vi "main v2.vi"() -> ()   [LabVIEW 2018]
uses:
  project/type defs/test keypad luster.ctl
  <vilib>/Instr/_visa.llb/VISA Configure Serial Port (Instr).vi
  type defs/Pelco_D_cmd.vi
  <vilib>/NI/Modbus Library/API/Wrapper/Create Serial Master.vi
  <vilib>/NI/Modbus Library/API/Master/Modbus Master.lvclass
  <vilib>/NI/Modbus Library/API/Wrapper/API Main.lvlib
panel:
  in  "autoFocus":bool
  out "Remote TILT":dbl format="%#_6f"
  out "Remote PAN":dbl format="%#_6f"
  in  "Client Closed":string="The client VI closed the connection."
  out "Reset status":bool
  in  "enable":bool=TRUE
  out "tilt":dbl
  out "pan":dbl
  in  "pan_right_limit(-10) 2":dbl=-20.0
  in  "pan left_limit(20) 2":dbl=20.0
  in  "tilt_down_limit(-10)":dbl=-10.0
  in  "tilt_up_limit(20)":dbl=20.0
  in  "delta tilt/sec":dbl=0.1 format="%#.13f"
  in  "delta pan/sec":dbl=0.1 format="%#.13f"
  out "launcher.compass":dbl format="%.1f"
  out "launcher.tilt":dbl format="%.1f"
  out "launcher.pan":dbl format="%.1f"
  out "magnification":string
  in  "get magnification":bool
  in  "cam default":bool
  in  "reset":bool
  out "Sync Status":bool
  out "keypad cmd":string
  out "CAM.tilt":dbl format="%#.2g"
  out "CAM.pan":dbl format="%.2f"
  in  "read tilt":bool
  in  "read pan":bool
  in  "close com":bool
  in  "open com":bool
  in  "stop":bool
  # "Launcher"
  # "Camera"
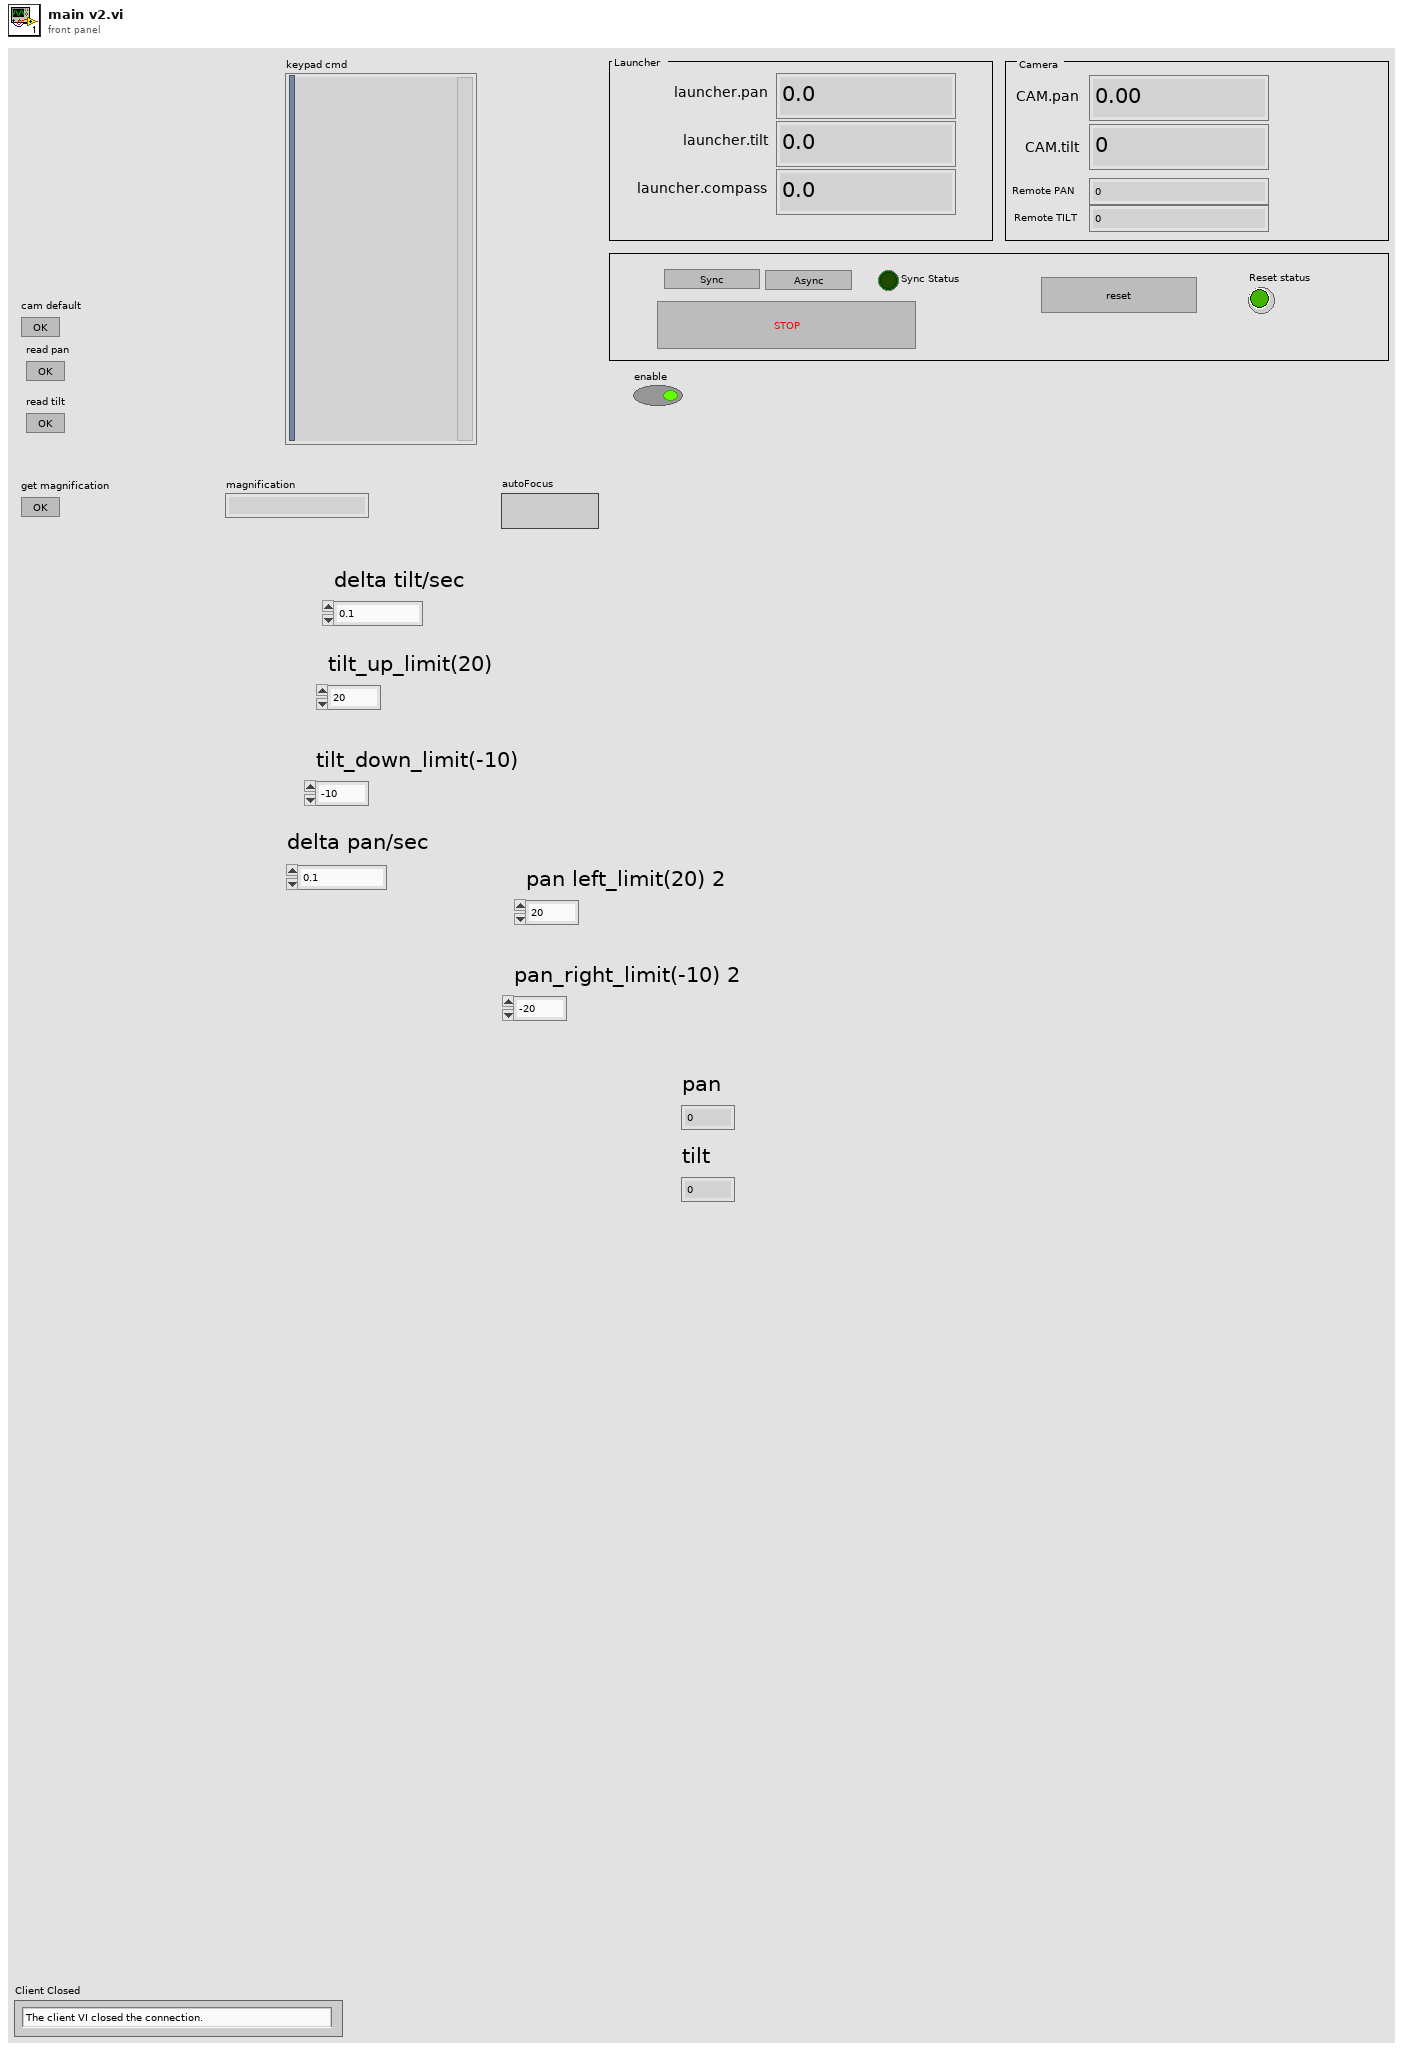
[diagram p1: front panel]
types:
  T1 = cluster{"launcher_pan":i16, "launcher_tilt":i16, "launcher_pan_leftLimit":i16, "launcher_pan_rightLimit":i16, "launcher_tilt_downLimit":i16, "launcher_tilt_upLimit":i16, "launcher_PLClink":i16, "launcher_PLCstatus":i16, "CAM_pan":i16, "CAM_tilt":i16}
  T2 = typedef "test keypad luster.ctl" = cluster{"cmd":string, "keypad cmd":variant}
  T3 = typedef "App Cluster.ctl" = cluster{"Hadware":cluster{"SPIM7.Keypad":refnum<visa-resource-name>, "SPIM7.CAM":refnum<visa-resource-name>, "PLC":refnum<visa-resource-name>, "Tester":refnum<visa-resource-name>, "ND3Comm":refnum<visa-resource-name>}, "Offset":cluster{"Pan":cluster{"a":dbl, "b":dbl}, "Tilt":cluster{"a":dbl, "b":dbl}}}
  T4 = cluster{"quit":refnum<user-event>, "read tilt":refnum<user-event>, "read pan":refnum<user-event>}
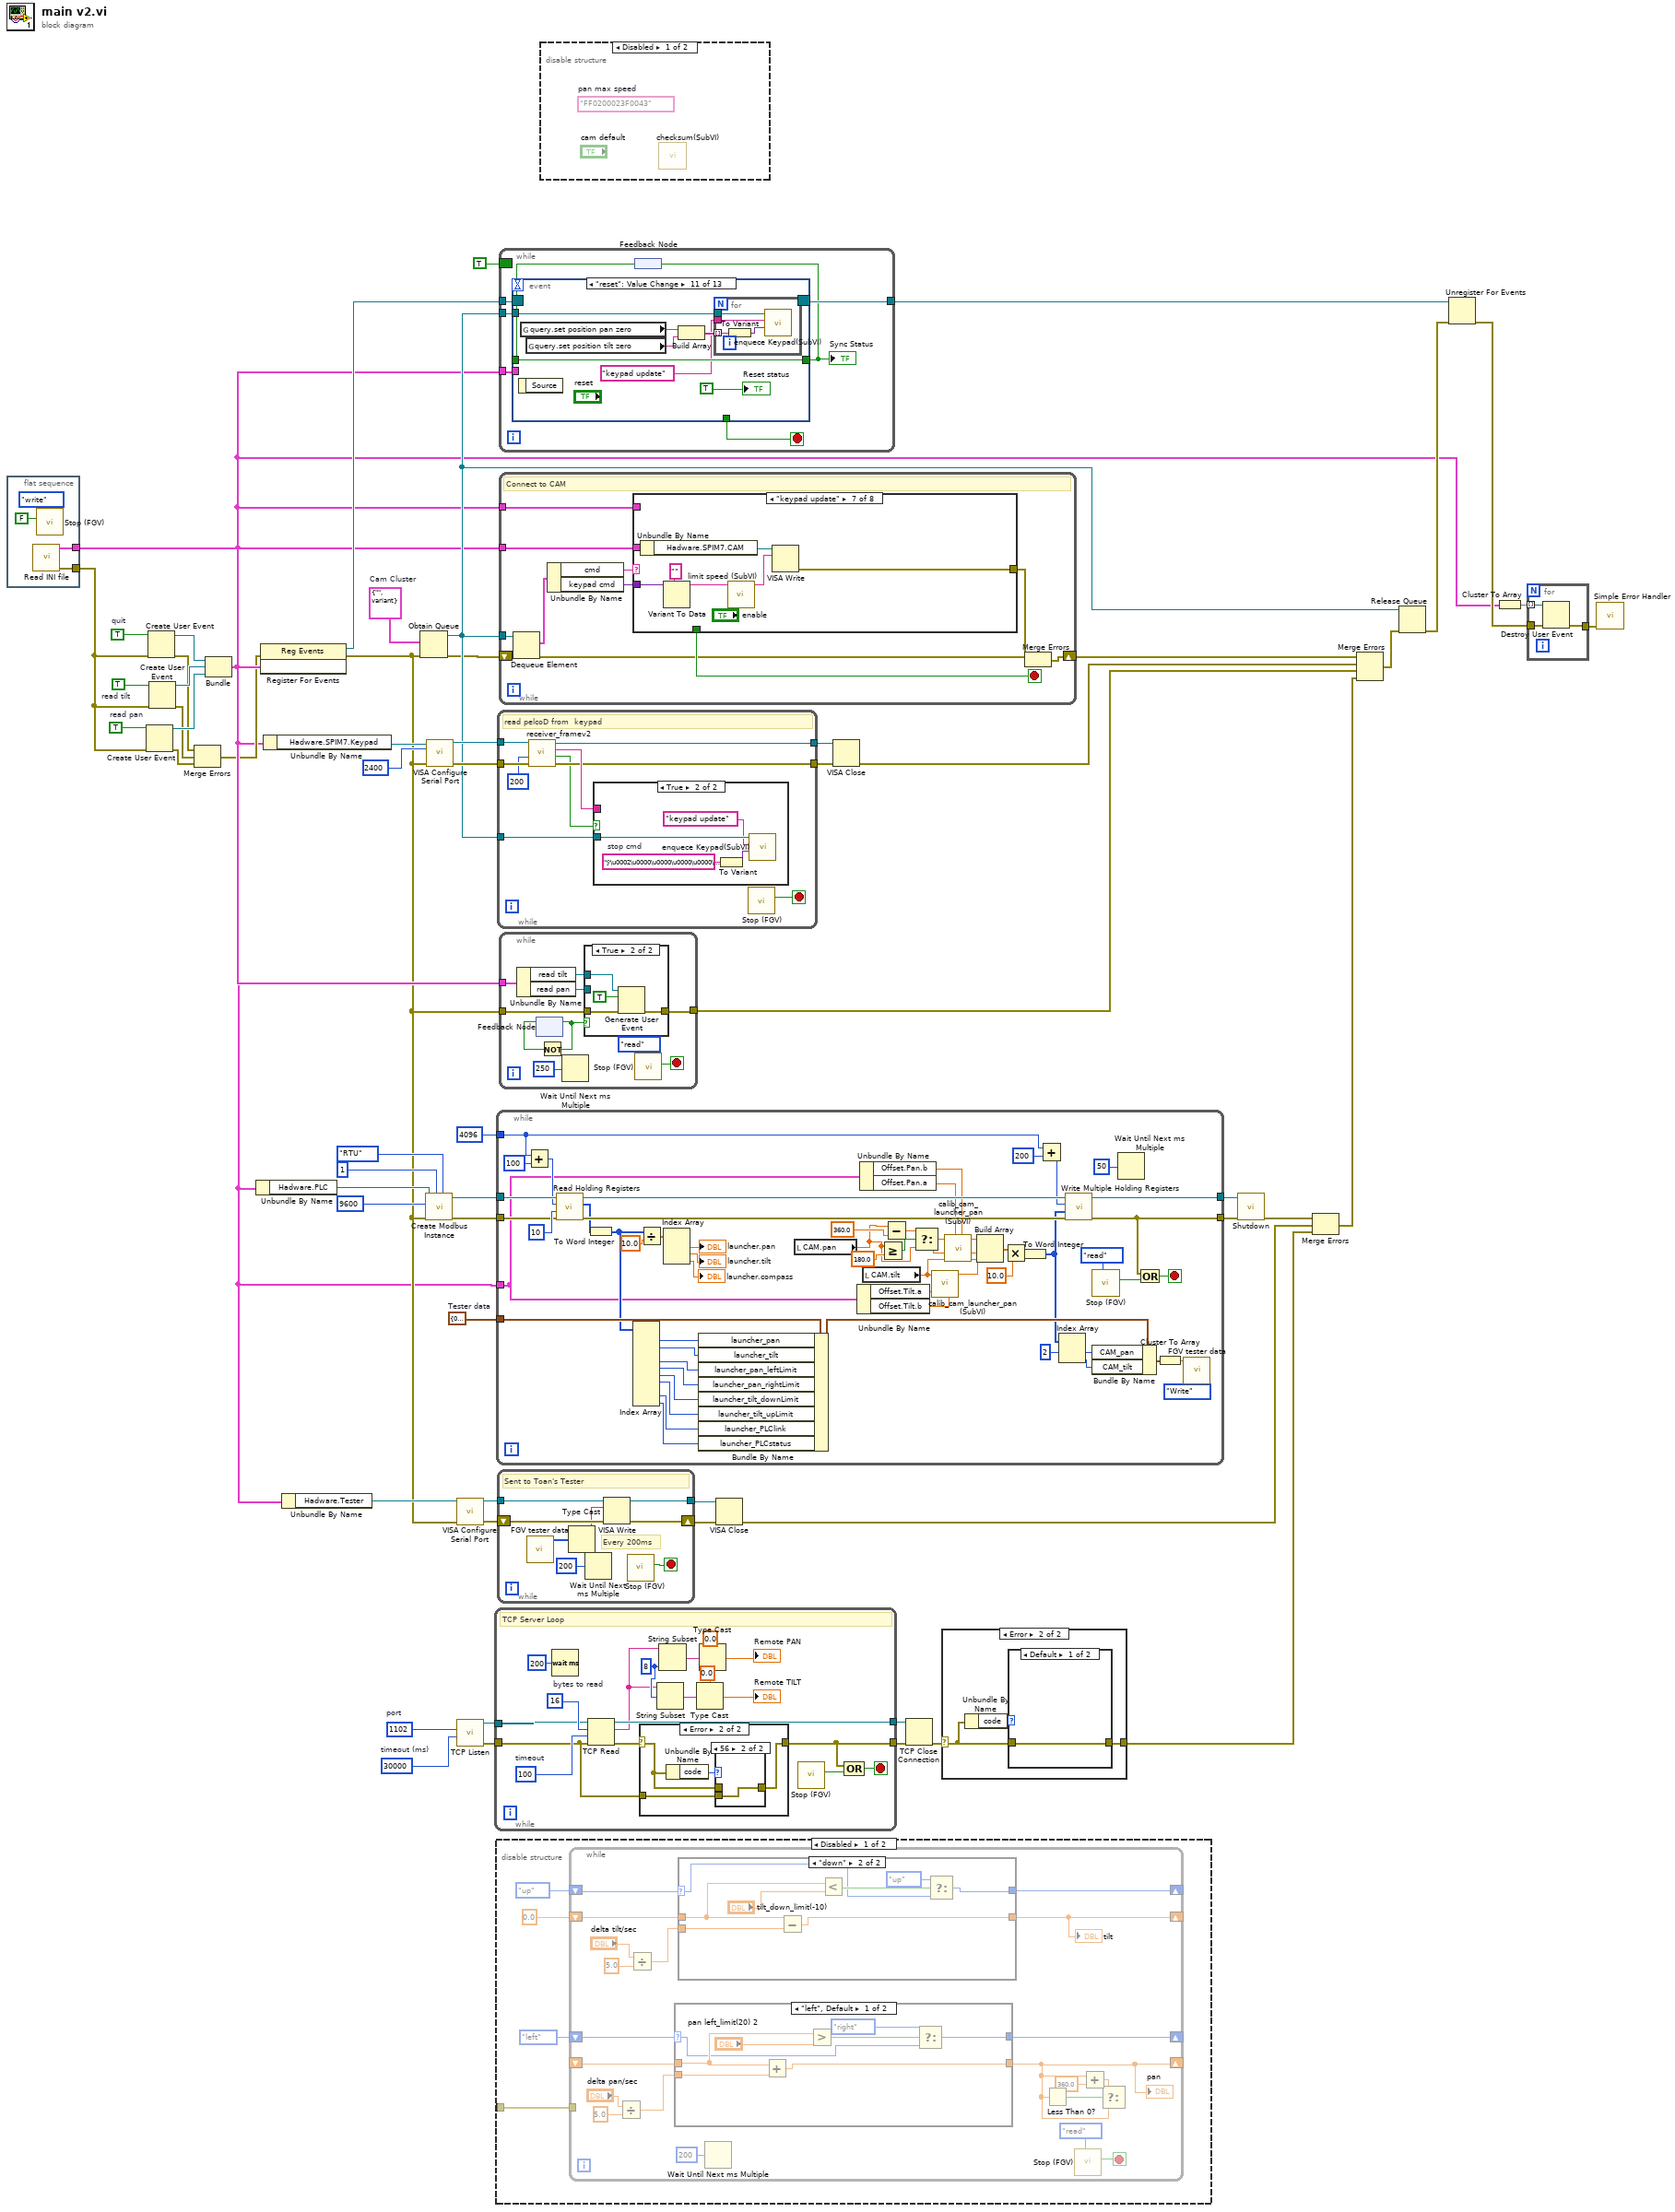
[diagram p0: block diagram]
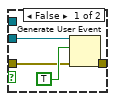
[diagram p2: hidden frame]
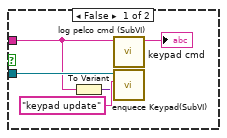
[diagram p3: hidden frame]
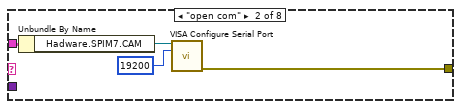
[diagram p5: hidden frame]
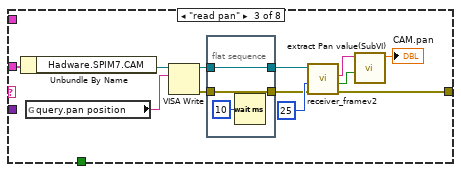
[diagram p6: hidden frame]
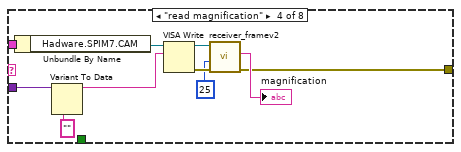
[diagram p7: hidden frame]
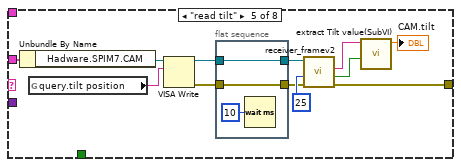
[diagram p8: hidden frame]
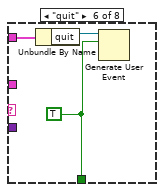
[diagram p9: hidden frame]
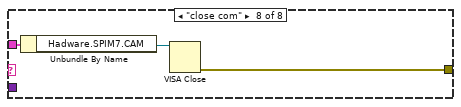
[diagram p10: hidden frame]
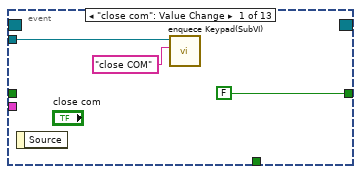
[diagram p11: hidden frame]
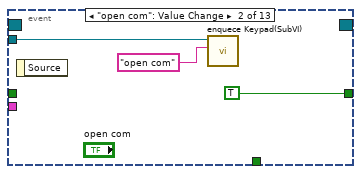
[diagram p12: hidden frame]
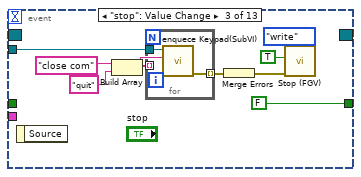
[diagram p13: hidden frame]
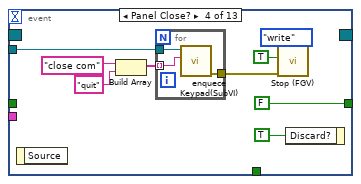
[diagram p14: hidden frame]
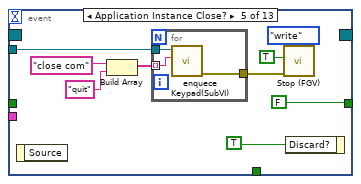
[diagram p15: hidden frame]
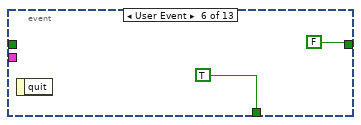
[diagram p16: hidden frame]
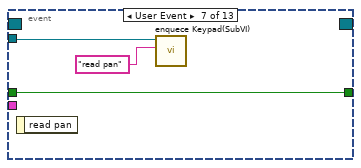
[diagram p17: hidden frame]
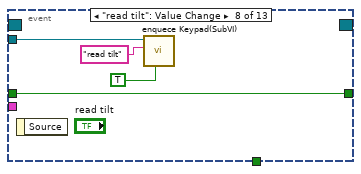
[diagram p18: hidden frame]
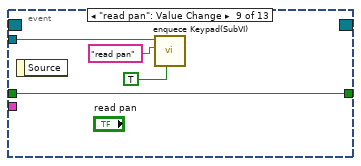
[diagram p19: hidden frame]
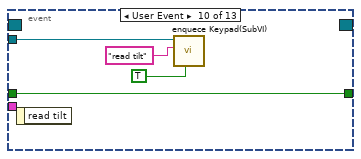
[diagram p20: hidden frame]
diagram:
  w27 = T1 {"launcher_pan"=0, "launcher_tilt"=0, "launcher_pan_leftLimit"=0, "launcher_pan_rightLimit"=0, "launcher_tilt_downLimit"=0, "launcher_tilt_upLimit"=0, "launcher_PLClink"=0, "launcher_PLCstatus"=0, "CAM_pan"=0, "CAM_tilt"=0}  # Tester data
  w13 = u16 1102  # port
  w14 = 30000  # timeout (ms)
  w47 = TRUE  # read pan
  w48 = TRUE  # read tilt
  w60 = TRUE  # quit
  w56 = T2 {"cmd"="", "keypad cmd"=variant(refnum<visa-resource-name> "")}  # Cam Cluster
  n1 = flat-sequence {
    tunnel: [w61] -> w41
    tunnel: [w62] -> w2
    frame #0 {
      n2 = call "Read INI file.vi"() -> ("error out"=w61:errorcluster, "App Cluster out"=w62:T3)  [unwired: 10 in]
      n3 = call "Stop (FGV).vi"("Enum(read)"=enum16{"write", "read"}."write" ("Enum"), "Stop in"=FALSE ("Boolean")) -> ()  [unwired: 8 in, 2 out]
    }
  }
  n4 = Create User Event(user event datatype=w47, error in=w41) -> (user event=w44:refnum<user-event>, error out=w8:errorcluster)
  n5 = Create User Event(user event datatype=w60, error in=w41) -> (user event=w46:refnum<user-event>, error out=w10:errorcluster)
  n6 = Create User Event(user event datatype=w48, error in=w41) -> (user event=w45:refnum<user-event>, error out=w9:errorcluster)
  n7 = Merge Errors(w10, w9, w8) -> (w7:errorcluster)
  n8 = Bundle("quit"=w46, "read tilt"=w45, "read pan"=w44) -> (w36:T4)  [unwired: 1 in]
  n9 = Unbundle By Name(w2) -> ("Hadware.PLC"=w5:refnum<visa-resource-name>)
  n10 = register-events(error in=w7, w36) -> (reference out=w59:refnum<event-registration>, error out=w3:errorcluster)  [unwired: 1 in]
  n11 = Unbundle By Name(w2) -> ("Hadware.SPIM7.Keypad"=w6:refnum<visa-resource-name>)
  n12 = Unbundle By Name(w2) -> ("Hadware.Tester"=w4:refnum<visa-resource-name>)
  n13 = Obtain Queue(element data type=w56, error in (no error)=w3) -> (queue out=w50:refnum<queue>, error out=w37:errorcluster)  [unwired: 3 in, 1 out]
  n14 = call-poly <vilib>:"Create Modbus Instance.vi"("serial type"=enum16{"RTU", "ASCII"}."RTU", "unit ID"=u8 1, "error in"=w3, "baud rate"=u32 9600, "VISA resource name"=w5) -> ("error out"=w30:errorcluster, "serial master instance"=w31:refnum<class "Modbus Master.lvclass">)  [unwired: 5 in]
  n15 = call-poly "VISA Configure Serial Port"("VISA resource name"=w6, "baud rate (9600)"=u32 2400, "error in (no error)"=w3) -> ("VISA resource name out"=w54:refnum<visa-resource-name>, "error out"=w53:errorcluster)  [unwired: 11 in]
  n16 = call-poly "VISA Configure Serial Port"("VISA resource name"=w4, "error in (no error)"=w3) -> ("VISA resource name out"=w26:refnum<visa-resource-name>, "error out"=w25:errorcluster)  [unwired: 12 in]
  n17 = call <vilib>:"TCP Listen.vi"("timeout ms (wait forever: -1)"=w14, "port"=w13) -> ("error out"=w15:errorcluster, "connection ID"=w16:refnum<k5>)  [unwired: 5 in, 3 out]
  n18 = while {
    tunnel: [w76] -> w18
    tunnel: [w79] -> w19
    tunnel: w16 -> [w75]
    tunnel: w15 -> [w74]
    stop <- w81 stop-if-true
    w70 = 8 ("length (rest)")
    w78 = 100  # timeout
    w80 = 16  # bytes to read
    # "TCP Server Loop"
    n19 = Wait (ms)(milliseconds to wait=u32 200) -> ()  [unwired: 1 out]
    n20 = TCP Read(connection ID=w75, bytes to read=w80, error in (no error)=w74, 9:w78) -> (connection ID out=w79:refnum<k5>, data out=w65:string, error out=w77:errorcluster)  [unwired: 1 out]
    n21 = case shown="Error" w77 {
      selector: w77 -> [w83 w86]
      tunnel: [w83 w84] -> w76
      tunnel: w74 -> [_ w85]
      frame No Error {
      }
      frame Error {
        n22 = Unbundle By Name(w86) -> ("code"=w87:i32)
        n23 = case shown="56" w87 {
          tunnel: w86 -> [w88 _]
          tunnel: w85 -> [_ w89]
          tunnel: [w88 w89] -> w84
          frame Default {
          }
          frame 56 {
          }
        }
      }
    }
    n24 = String Subset(string=w65, offset (0)=w70) -> (substring=w68:string)  [unwired: 1 in]
    n25 = String Subset(string=w65, length (rest)=w70) -> (substring=w72:string)  [unwired: 1 in]
    n26 = Type Cast(type=0.0, x=w68) -> (*(type *) &x=→"Remote TILT":dbl)
    n27 = Type Cast(type=0.0, x=w72) -> (*(type *) &x=→"Remote PAN":dbl)
    n28 = call "Stop (FGV).vi"() -> ("Stop out"=w66:bool)  [unwired: 10 in, 1 out]
    n29 = Compound Arithmetic op=OR(w76, w66) -> (w81:bool)
  }
  n30 = while {
    tunnel: u16 4096 -> [w139]
    tunnel: w31 -> [w145]
    tunnel: w30 -> [w141]
    tunnel: [w131] -> w28
    tunnel: [w133] -> w29
    tunnel: w27 -> [w113]
    tunnel: w2 -> [w92]
    stop <- w129 stop-if-true
    n31 = Add(x=w139, y=u16 100) -> (x+y=w143:u16)
    n32 = call-dynamic "Read Holding Registers.vi"("error in"=w141, "number of inputs"=u16 10, "starting address"=w143, "Modbus master in"=w145) -> ("error out"=w134:errorcluster, "register values"=w128:u16[], "Modbus master out"=w136:refnum<class "Modbus Master.lvclass">)  [unwired: 5 in]
    n33 = To Word Integer(number=w128) -> (16bit integer=w111:i16[])
    n34 = Index Array(array=w111) -> (element #1=w110:i16, element #2=w109:i16, element #4=w108:i16, element #5=w107:i16, element #6=w106:i16, element #7=w105:i16, element #9=w104:i16, element #10=w103:i16)  [unwired: 10 in, 2 out]
    n35 = Divide(x=w111, y=10.0) -> (x/y=w124:dbl[])
    n36 = Index Array(array=w124) -> (element #1=→"launcher.pan":dbl, element #2=→"launcher.tilt":dbl, element #3=→"launcher.compass":dbl)  [unwired: 3 in]
    n37 = Bundle By Name(cluster=w113, "launcher_pan"=w110, "launcher_tilt"=w109, "launcher_pan_leftLimit"=w108, "launcher_pan_rightLimit"=w107, "launcher_tilt_downLimit"=w106, "launcher_tilt_upLimit"=w105, "launcher_PLClink"=w104, "launcher_PLCstatus"=w103) -> (w102:T1)
    n38 = local read "CAM.pan"() -> (w118:dbl)
    n39 = Unbundle By Name(w92) -> ("Offset.Tilt.a"=w91:dbl, "Offset.Tilt.b"=w90:dbl)
    n40 = Unbundle By Name(w92) -> ("Offset.Pan.b"=w94:dbl, "Offset.Pan.a"=w93:dbl)
    n41 = local read "CAM.tilt"() -> (w114:dbl)
    n42 = Greater Or Equal?(x=w118, y=180.0) -> (x >= y?=w121:bool)
    n43 = Subtract(x=w118, y=360.0) -> (x-y=w120:dbl)
    n44 = Select(t=w120, s=w121, f=w118) -> (s? t:f=w115:dbl)
    n45 = call "calib_cam_launcher_pan (SubVI).vi"("b"=w90, "a"=w91, "x"=w114) -> ("y"=w116:dbl)  [unwired: 8 in]
    n46 = call "calib_cam_launcher_pan (SubVI).vi"("b"=w94, "a"=w93, "x"=w115) -> ("y"=w117:dbl)  [unwired: 8 in]
    n47 = Build Array(w117, w116, w115, w114) -> (w138:dbl[])
    n48 = Multiply(x=w138, y=10.0) -> (x*y=w112:dbl[])
    n49 = To Word Integer(number=w112) -> (16bit integer=w101:i16[])
    n50 = Add(x=w139, y=u16 200) -> (x+y=w135:u16)
    n51 = Index Array(array=w101, index #1=2 ("index")) -> (element #1=w99:i16, element #2=w98:i16)  [unwired: 1 in]
    n52 = call-dynamic "Write Multiple Holding Registers.vi"("error in"=w134, "registers to write"=w101, "starting address"=w135, "Modbus master in"=w136) -> ("error out"=w131:errorcluster, "Modbus master out"=w133:refnum<class "Modbus Master.lvclass">)  [unwired: 6 in]
    n53 = Bundle By Name(cluster=w102, "CAM_pan"=w99, "CAM_tilt"=w98) -> (w96:T1)
    n54 = call "Stop (FGV).vi"("Enum(read)"=enum16{"write", "read"}."read" ("Enum")) -> ("Stop out"=w130:bool)  [unwired: 9 in, 1 out]
    n55 = Wait Until Next ms Multiple(millisecond multiple=u32 50) -> ()  [unwired: 1 out]
    n56 = Or(x=w131, y=w130) -> (x .or. y?=w129:bool)
    n57 = Cluster To Array(cluster=w96) -> (array=w95:i16[])
    n58 = call "FGV tester data.vi"("Enum(read)"=enum16{"Write", "Read"}."Write" ("Enum"), "data in"=w95) -> ()  [unwired: 9 in, 1 out]
  }
  n59 = disable-structure shown="Disabled" {
    disable-tunnel: _ -> [w147 _]
    frame Disabled {
      n60 = while {
        shift-right: [w162] -> _
        shift-left: 0.0 -> [w166]
        shift-right: [w157] -> _
        shift-left: _ -> [w164]
        shift-right: [w165] -> _
        shift-left: enum16{"up", "down"}."up" -> [w167]
        shift-right: [w161] -> _
        shift-left: enum16{"left", "right"}."left" -> [w163]
        tunnel: w147 -> [_]
        stop <- w168 stop-if-true
        n61 = Divide(x="delta pan/sec", y=5.0) -> (x/y=w154:dbl)
        n62 = Divide(x="delta tilt/sec", y=5.0) -> (x/y=w151:dbl)
        n63 = case shown="\"left\", Default" w163 {
          selector: w163 -> [w173 w181]
          tunnel: w154 -> [w178 w186]
          tunnel: w164 -> [w176 w184]
          tunnel: [w177 w179] -> w157
          tunnel: [w172 w182] -> w161
          frame "left", Default {
            n64 = Add(x=w176, y=w178) -> (x+y=w177:dbl)
            n65 = Greater?(x=w176, y="pan left_limit(20) 2") -> (0:w174:bool)
            n66 = Select(t=enum16{"left", "right"}."right", s=w174, f=w173) -> (s? t:f=w172:enum16{"left", "right"})
          }
          frame "right" {
            n67 = Subtract(x=w184, y=w186) -> (x-y=w179:dbl)
            n68 = Less?(x=w184, y="pan_right_limit(-10) 2") -> (x < y?=w183:bool)
            n69 = Select(t=enum16{"left", "right"}."left", s=w183, f=w181) -> (s? t:f=w182:enum16{"left", "right"})
          }
        }
        "pan" <- w157
        n70 = case shown="\"down\"" w167 {
          selector: w167 -> [w188 w195]
          tunnel: w151 -> [w194 w202]
          tunnel: w166 -> [w192 w199]
          tunnel: [w193 w201] -> w162
          tunnel: [w187 w197] -> w165
          frame "up", Default {
            n71 = Add(x=w192, y=w194) -> (x+y=w193:dbl)
            n72 = Greater?(x=w192, y="tilt_up_limit(20)") -> (0:w190:bool)
            n73 = Select(t=enum16{"up", "down"}."down", s=w190, f=w188) -> (s? t:f=w187:enum16{"up", "down"})
          }
          frame "down" {
            n74 = Subtract(x=w199, y=w202) -> (x-y=w201:dbl)
            n75 = Less?(x=w199, y="tilt_down_limit(-10)") -> (x < y?=w198:bool)
            n76 = Select(t=enum16{"up", "down"}."up", s=w198, f=w195) -> (s? t:f=w197:enum16{"up", "down"})
          }
        }
        "tilt" <- w162
        n77 = Wait Until Next ms Multiple(millisecond multiple=u32 200) -> ()  [unwired: 1 out]
        n78 = Less Than 0?(x=w157) -> (x < 0?=w160:bool)
        n79 = call "Stop (FGV).vi"("Enum(read)"=enum16{"write", "read"}."read" ("Enum")) -> ("Stop out"=w168:bool)  [unwired: 9 in, 1 out]
        n80 = Add(x=w157, y=360.0) -> (x+y=w158:dbl)
        n81 = Select(t=w158, s=w160, f=w157) -> ()  [unwired: 1 out]
      }
    }
    frame Enabled {
    }
  }
  n82 = while {
    tunnel: w54 -> [w211]
    tunnel: w53 -> [w210]
    tunnel: [w208] -> w52
    tunnel: [w207] -> w51
    tunnel: w50 -> [w205]
    stop <- w204 stop-if-true
    # "read pelcoD from  keypad"
    n83 = call "receiver_framev2.vi"("error in (no error)"=w210, "Timeout(100ms)"=u32 200, "Visa In"=w211) -> ("error out"=w208:errorcluster, "TimeOut?"=w206:bool, "response"=w209:string, "Visa out"=w207:refnum<visa-resource-name>)  [unwired: 5 in]
    n84 = case shown="True" w206 {
      tunnel: w209 -> [w213 _]
      tunnel: w205 -> [w216 w220]
      frame False {
        n85 = To Variant(anything=w213) -> (Variant=w214:variant)
        n86 = call "log pelco cmd (SubVI).vi"("String"=w213) -> ("Cam rcv"=→"keypad cmd":string)  [unwired: 10 in]
        n87 = call "enquece Keypad(SubVI).vi"("keypad cmd"=w214, "cmd"="keypad update", "Queue in"=w216) -> ()  [unwired: 7 in, 2 out]
      }
      frame True {
        w218 = "ÿ\u0002\u0000\u0000\u0000\u0000\u0002"  # stop cmd
        n88 = To Variant(anything=w218) -> (Variant=w217:variant)
        n89 = call "enquece Keypad(SubVI).vi"("keypad cmd"=w217, "cmd"="keypad update", "Queue in"=w220) -> ()  [unwired: 7 in, 2 out]
      }
    }
    n90 = call "Stop (FGV).vi"() -> ("Stop out"=w204:bool)  [unwired: 10 in, 1 out]
  }
  n91 = while {
    tunnel: w26 -> [w228]
    shift-right: [w225] -> w24
    shift-left: w25 -> [w227]
    tunnel: [w224] -> w23
    stop <- w226 stop-if-true
    # "Every 200ms"
    # "Sent to Toan's Tester"
    n92 = call "FGV tester data.vi"() -> ("data in 2"=w222:i16[])  [unwired: 11 in]
    n93 = Type Cast(x=w222) -> (*(type *) &x=w221:string)  [unwired: 1 in]
    n94 = Wait Until Next ms Multiple(millisecond multiple=u32 200) -> ()  [unwired: 1 out]
    n95 = VISA Write(VISA resource name=w228, write buffer=w221, error in (no error)=w227) -> (VISA resource name out=w224:refnum<visa-resource-name>, error out=w225:errorcluster)  [unwired: 1 out]
    n96 = call "Stop (FGV).vi"() -> ("Stop out"=w226:bool)  [unwired: 10 in, 1 out]
  }
  n97 = while {
    tunnel: w50 -> [w234]
    tunnel: w59 -> [w235]
    tunnel: [w233] -> w58
    border: TRUE -> [_]
    tunnel: w36 -> [w229]
    stop <- w232 stop-if-true
    n98 = feedback #1() -> (w230:bool)
    n99 = event shown="[10] \"reset\": Value Change" {
      selector: w235 -> [_ _ _ _ _ _ _ _ _ _ _ _ _]
      dyn-events: [_ _ _ _ _ _ _ _ _ _ _ _ _] -> w233
      timeout: _ -> [_ _ _ _ _ _ _ _ _ _ _ _ _]
      tunnel: w234 -> [w238 w241 w250 w262 w274 _ w282 w286 w289 w293 w301 w314 w319]
      tunnel: [_ _ _ _ _ TRUE _ _ _ _ _ _ _] -> w232
      tunnel: [FALSE TRUE FALSE FALSE FALSE FALSE w281 w285 w290 w294 w299 w315 w320] -> w231
      tunnel: w230 -> [_ _ _ _ _ _ w281 w285 w290 w294 w299 w315 w320]
      tunnel: w229 -> [_ _ _ _ _ _ _ _ _ _ _ _ _]
      event "close com": Value Change {
        n100 = event-data() -> ()  [unwired: 1 in, 1 out]
        n101 = call "enquece Keypad(SubVI).vi"("cmd"="close COM", "Queue in"=w238) -> ()  [unwired: 8 in, 2 out]
      }
      event "open com": Value Change {
        n102 = event-data() -> ()  [unwired: 1 in, 1 out]
        n103 = call "enquece Keypad(SubVI).vi"("cmd"="open com" ("element"), "Queue in"=w241) -> ()  [unwired: 8 in, 2 out]
      }
      event "stop": Value Change {
        n104 = event-data() -> ()  [unwired: 1 in, 1 out]
        n105 = Build Array("close com", "quit") -> (w245:string[])
        n106 = for {
          tunnel: w245 -> [w251] mode=indexing
          tunnel: w250 -> [w253]
          tunnel: [w252] -> w243 mode=indexing
          n107 = call "enquece Keypad(SubVI).vi"("cmd"=w251, "Queue in"=w253) -> ("error out"=w252:errorcluster)  [unwired: 8 in, 1 out]
        }
        n108 = Merge Errors(w243) -> (w242:errorcluster)
        n109 = call "Stop (FGV).vi"("Enum(read)"=enum16{"write", "read"}."write" ("Enum"), "error in (no error)"=w242, "Stop in"=TRUE ("Boolean")) -> ()  [unwired: 7 in, 2 out]
      }
      event Panel Close? {
        n110 = event-data() -> ()  [unwired: 1 in, 1 out]
        n111 = Build Array("close com", "quit") -> (w257:string[])
        n112 = for {
          tunnel: w257 -> [w263] mode=indexing
          tunnel: w262 -> [w265]
          tunnel: [w264] -> w255
          n113 = call "enquece Keypad(SubVI).vi"("cmd"=w263, "Queue in"=w265) -> ("error out"=w264:errorcluster)  [unwired: 8 in, 1 out]
        }
        n114 = call "Stop (FGV).vi"("Enum(read)"=enum16{"write", "read"}."write" ("Enum"), "error in (no error)"=w255, "Stop in"=TRUE ("Boolean")) -> ()  [unwired: 7 in, 2 out]
        n115 = event-data("Discard?"=TRUE) -> ()  [unwired: 1 in, 1 out]
      }
      event Application Instance Close? {
        n116 = event-data() -> ()  [unwired: 1 in, 1 out]
        n117 = Build Array("close com", "quit") -> (w269:string[])
        n118 = for {
          tunnel: w269 -> [w275] mode=indexing
          tunnel: w274 -> [w277]
          tunnel: [w276] -> w267
          n119 = call "enquece Keypad(SubVI).vi"("cmd"=w275, "Queue in"=w277) -> ("error out"=w276:errorcluster)  [unwired: 8 in, 1 out]
        }
        n120 = call "Stop (FGV).vi"("Enum(read)"=enum16{"write", "read"}."write" ("Enum"), "error in (no error)"=w267, "Stop in"=TRUE ("Boolean")) -> ()  [unwired: 7 in, 2 out]
        n121 = event-data("Discard?"=TRUE) -> ()  [unwired: 1 in, 1 out]
      }
      event User Event {
        n122 = event-data() -> ()  [unwired: 1 in, 1 out]
      }
      event User Event {
        n123 = event-data() -> ()  [unwired: 1 in, 1 out]
        n124 = call "enquece Keypad(SubVI).vi"("cmd"="read pan", "Queue in"=w282) -> ()  [unwired: 8 in, 2 out]
      }
      event "read tilt": Value Change {
        n125 = event-data() -> ()  [unwired: 1 in, 1 out]
        n126 = call "enquece Keypad(SubVI).vi"("priority enquece"=TRUE, "cmd"="read tilt", "Queue in"=w286) -> ()  [unwired: 7 in, 2 out]
      }
      event "read pan": Value Change {
        n127 = event-data() -> ()  [unwired: 1 in, 1 out]
        n128 = call "enquece Keypad(SubVI).vi"("priority enquece"=TRUE, "cmd"="read pan", "Queue in"=w289) -> ()  [unwired: 7 in, 2 out]
      }
      event User Event {
        n129 = event-data() -> ()  [unwired: 1 in, 1 out]
        n130 = call "enquece Keypad(SubVI).vi"("priority enquece"=TRUE, "cmd"="read tilt", "Queue in"=w293) -> ()  [unwired: 7 in, 2 out]
      }
      event "reset": Value Change {
        n131 = event-data() -> ()  [unwired: 1 in, 1 out]
        n132 = global read "Pelco_D_cmd.vi" "query.set position pan zero"() -> (w298:string)
        n133 = global read "Pelco_D_cmd.vi" "query.set position tilt zero"() -> (w297:string)
        n134 = Build Array(w298, w297) -> (w300:string[])
        n135 = for {
          tunnel: w301 -> [w305]
          tunnel: w300 -> [w304] mode=indexing
          tunnel: "keypad update" ("cmd") -> [w302]
          n136 = To Variant(anything=w304) -> (Variant=w303:variant)
          n137 = call "enquece Keypad(SubVI).vi"("keypad cmd"=w303, "cmd"=w302, "Queue in"=w305) -> ()  [unwired: 7 in, 2 out]
        }
        "Reset status" <- TRUE
      }
      event "autoFocus": Value Change {
        n138 = event-data() -> ()  [unwired: 1 in, 1 out]
        n139 = feedback #2(FALSE) -> (w311:bool)
        n140 = Not(x=w311) -> (.not. x?=w309:bool)
        n141 = feedback-in #2(w309) -> ()
        n142 = Select(t="ÿ\u0002\u0000+\u0000\u0000\u0000-", s=w309, f="ÿ\u0002\u0000+\u0000\u0001\u0000.") -> (s? t:f=w306:string)
        n143 = To Variant(anything=w306) -> (Variant=w312:variant)
        n144 = call "enquece Keypad(SubVI).vi"("keypad cmd"=w312, "cmd"="keypad update", "Queue in"=w314) -> ()  [unwired: 7 in, 2 out]
      }
      event "get magnification": Value Change {
        n145 = event-data() -> ()  [unwired: 1 in, 1 out]
        n146 = global read "Pelco_D_cmd.vi" "query. query magnification"() -> (w317:string)
        n147 = To Variant(anything=w317) -> (Variant=w318:variant)
        n148 = call "enquece Keypad(SubVI).vi"("keypad cmd"=w318, "cmd"="keypad update", "Queue in"=w319) -> ()  [unwired: 7 in, 2 out]
      }
    }
    "Sync Status" <- w231
    n149 = feedback-in #1(w231) -> ()
  }
  n150 = while {
    tunnel: w50 -> [w330]
    tunnel: w36 -> [w328]
    tunnel: w2 -> [w325]
    shift-right: [w323] -> w11
    shift-left: w37 -> [w331]
    stop <- w327 stop-if-true
    # "Connect to CAM"
    n151 = Dequeue Element(queue=w330, error in (no error)=w331) -> (element=w326:T2, error out=w324:errorcluster)  [unwired: 1 in, 2 out]
    n152 = Unbundle By Name(w326) -> ("cmd"=w329:string, "keypad cmd"=w322:variant)
    n153 = case shown="\"keypad update\"" w329 {
      tunnel: w325 -> [_ w332 w347 w355 w372 _ w384 w388]
      tunnel: w328 -> [_ _ _ _ _ w377 _ _]
      tunnel: [_ _ _ _ _ w378 _ _] -> w327
      tunnel: [_ w334 w342 w352 w367 _ w383 w387] -> w321
      tunnel: w322 -> [_ _ _ w351 _ _ w379 _]
      frame "False", Default {
      }
      frame "open com" {
        n154 = Unbundle By Name(w332) -> ("Hadware.SPIM7.CAM"=w333:refnum<visa-resource-name>)
        n155 = call-poly "VISA Configure Serial Port"("VISA resource name"=w333, "baud rate (9600)"=u32 19200) -> ("error out"=w334:errorcluster)  [unwired: 12 in, 1 out]
      }
      frame "read pan" {
        n156 = Unbundle By Name(w347) -> ("Hadware.SPIM7.CAM"=w336:refnum<visa-resource-name>)
        n157 = global read "Pelco_D_cmd.vi" "query.pan position"() -> (w343:string)
        n158 = VISA Write(VISA resource name=w336, write buffer=w343) -> (VISA resource name out=w340:refnum<visa-resource-name>, error out=w338:errorcluster)  [unwired: 1 in, 1 out]
        n159 = flat-sequence {
          tunnel: [w350] -> w341
          tunnel: w340 -> [w350]
          tunnel: [w349] -> w339
          tunnel: w338 -> [w349]
          frame #0 {
            n160 = Wait (ms)(milliseconds to wait=u32 10) -> ()  [unwired: 1 out]
          }
        }
        n161 = call "receiver_framev2.vi"("error in (no error)"=w339, "Timeout(100ms)"=u32 25, "Visa In"=w341) -> ("error out"=w342:errorcluster, "TimeOut?"=w345:bool, "response"=w346:string)  [unwired: 5 in, 1 out]
        n162 = call "extract Pan value(SubVI).vi"("TimeOut"=w345, "response"=w346) -> ("pan angle"=→"CAM.pan":dbl)  [unwired: 8 in, 1 out]
      }
      frame "read magnification" {
        n163 = Unbundle By Name(w355) -> ("Hadware.SPIM7.CAM"=w360:refnum<visa-resource-name>)
        n164 = Variant To Data(type="", Variant=w351) -> (data=w353:string)  [unwired: 1 in, 1 out]
        n165 = VISA Write(VISA resource name=w360, write buffer=w353) -> (VISA resource name out=w359:refnum<visa-resource-name>, error out=w358:errorcluster)  [unwired: 1 in, 1 out]
        n166 = call "receiver_framev2.vi"("error in (no error)"=w358, "Timeout(100ms)"=u32 25, "Visa In"=w359) -> ("error out"=w352:errorcluster, "response"=→"magnification":string)  [unwired: 5 in, 2 out]
      }
      frame "read tilt" {
        n167 = Unbundle By Name(w372) -> ("Hadware.SPIM7.CAM"=w361:refnum<visa-resource-name>)
        n168 = global read "Pelco_D_cmd.vi" "query.tilt position"() -> (w368:string)
        n169 = VISA Write(VISA resource name=w361, write buffer=w368) -> (VISA resource name out=w365:refnum<visa-resource-name>, error out=w363:errorcluster)  [unwired: 1 in, 1 out]
        n170 = flat-sequence {
          tunnel: [w374] -> w366
          tunnel: w365 -> [w374]
          tunnel: [w373] -> w364
          tunnel: w363 -> [w373]
          frame #0 {
            n171 = Wait (ms)(milliseconds to wait=u32 10) -> ()  [unwired: 1 out]
          }
        }
        n172 = call "receiver_framev2.vi"("error in (no error)"=w364, "Timeout(100ms)"=u32 25, "Visa In"=w366) -> ("error out"=w367:errorcluster, "TimeOut?"=w370:bool, "response"=w371:string)  [unwired: 5 in, 1 out]
        n173 = call "extract Tilt value(SubVI).vi"("Time out?"=w370, "Pelco-D response"=w371) -> ("tilt1"=→"CAM.tilt":dbl)  [unwired: 8 in, 1 out]
      }
      frame "quit" {
        w378 = TRUE ("event data")
        n174 = Unbundle By Name(w377) -> ("quit"=w376:refnum<user-event>)
        n175 = Generate User Event(user event=w376, event data cluster=w378) -> ()  [unwired: 2 in, 2 out]
      }
      frame "keypad update" {
        n176 = Unbundle By Name(w384) -> ("Hadware.SPIM7.CAM"=w385:refnum<visa-resource-name>)
        n177 = Variant To Data(type="", Variant=w379) -> (data=w382:string)  [unwired: 1 in, 1 out]
        n178 = call "limit speed (SubVI).vi"("enable"="enable", "keypad cmd"=w382) -> ("keypad cmd  out"=w381:string)  [unwired: 9 in]
        n179 = VISA Write(VISA resource name=w385, write buffer=w381) -> (error out=w383:errorcluster)  [unwired: 1 in, 2 out]
      }
      frame "close com" {
        n180 = Unbundle By Name(w388) -> ("Hadware.SPIM7.CAM"=w389:refnum<visa-resource-name>)
        n181 = VISA Close(VISA resource name=w389) -> (error out=w387:errorcluster)  [unwired: 1 in]
      }
    }
    n182 = Merge Errors(w324, w321) -> (w323:errorcluster)
  }
  n183 = while {
    tunnel: w36 -> [w397]
    tunnel: w3 -> [w396]
    tunnel: [w395] -> w39
    stop <- w398 stop-if-true
    n184 = Unbundle By Name(w397) -> ("read tilt"=w393:refnum<user-event>, "read pan"=w392:refnum<user-event>)
    n185 = feedback #3() -> (w391:bool)  [unwired: 1 in]
    n186 = Not(x=w391) -> (.not. x?=w390:bool)
    n187 = feedback-in #3(w390) -> ()
    n188 = Wait Until Next ms Multiple(millisecond multiple=u32 250) -> ()  [unwired: 1 out]
    n189 = case shown="True" w390 {
      tunnel: w393 -> [_ w407]
      tunnel: w392 -> [w403 _]
      tunnel: w396 -> [w401 w406]
      tunnel: [w400 w405] -> w395
      frame False {
        n190 = Generate User Event(user event=w403, event data cluster=TRUE ("event data"), error in=w401) -> (error out=w400:errorcluster)  [unwired: 1 in, 1 out]
      }
      frame True {
        n191 = Generate User Event(user event=w407, event data cluster=TRUE ("event data"), error in=w406) -> (error out=w405:errorcluster)  [unwired: 1 in, 1 out]
      }
    }
    n192 = call "Stop (FGV).vi"("Enum(read)"=enum16{"write", "read"}."read" ("Enum")) -> ("Stop out"=w398:bool)  [unwired: 9 in, 1 out]
  }
  n193 = disable-structure shown="Disabled" {
    frame Disabled {
      (unwired) "FF0200023F0043"  # pan max speed
      n194 = call "checksum(SubVI).vi"() -> ()  [unwired: 11 in, 1 out]
    }
    frame Enabled {
    }
  }
  n195 = VISA Close(VISA resource name=w23, error in (no error)=w24) -> (error out=w22:errorcluster)
  n196 = VISA Close(VISA resource name=w51, error in (no error)=w52) -> (error out=w38:errorcluster)
  n197 = TCP Close Connection(connection ID=w19, error in (no error)=w18) -> (error out=w17:errorcluster)  [unwired: 2 out]
  n198 = case shown="Error" w17 {
    selector: w17 -> [w408 w410]
    tunnel: [w408 w409] -> w1
    frame No Error {
    }
    frame Error {
      n199 = Unbundle By Name(w410) -> ("code"=w411:i32)
      n200 = case shown="Default" w411 {
        tunnel: w410 -> [w412 _]
        tunnel: [w412 w414] -> w409
        frame Default {
        }
        frame 62, 64, 66 {
          w414 = errorcluster {"status"=FALSE, "code"=0, "source"=""}  # No error
          n201 = One Button Dialog(message="Client Closed") -> ()  [unwired: 1 in, 1 out]
        }
      }
    }
  }
  n202 = call-dynamic "Shutdown.vi"("error in"=w28, "Modbus master in"=w29) -> ("error out"=w21:errorcluster)  [unwired: 9 in]
  n203 = Merge Errors(w21, w22, w1) -> (w20:errorcluster)
  n204 = Merge Errors(w11, w38, w39, w20) -> (w40:errorcluster)
  n205 = Release Queue(queue=w50, error in (no error)=w40) -> (error out=w49:errorcluster)  [unwired: 1 in, 2 out]
  n206 = Unregister For Events(event registration refnum=w58, error in=w49) -> (error out=w57:errorcluster)
  n207 = Cluster To Array(cluster=w36) -> (array=w43:refnum<user-event>[])
  n208 = for {
    tunnel: w57 -> [w417]
    tunnel: w43 -> [w416] mode=indexing
    tunnel: [w415] -> w42
    n209 = Destroy User Event(user event=w416, error in=w417) -> (error out=w415:errorcluster)
  }
  n210 = call <vilib>:"Simple Error Handler.vi"("error in (no error)"=w42) -> ()  [unwired: 4 in, 5 out]
